vi "Reproductor de musica.vi"() -> ()   [LabVIEW 2023]
uses:
  <vilib>/Analysis/3filter.llb/Filter Passband Type.ctl
  <vilib>/express/express analysis/Spectral/Block/exnSpectralBlock spectral measurements power poly.vi
  <vilib>/express/express analysis/Spectral/XNode/ExpressSpectralMeasurementsBlockNode.xnode
  <vilib>/measure/mamon.llb/Waveform Peak Detection for 1 Chan.vi
  <vilib>/express/express analysis/Spectral/Block/exnSpectralBlock spectral measurements power WFM.vi
  <vilib>/Analysis/3filter.llb/Butterworth Filter (DBL).vi
  <vilib>/Waveform/WDTOps.llb/WDT Get Waveform Subset DBL.vi
  <vilib>/Waveform/WDTOps.llb/WDT Number of Waveform Samples DBL.vi
  <vilib>/Waveform/WDTOps.llb/WDT Waveform Duration DBL.vi
  <vilib>/Analysis/NI_AALBase.lvlib
  <vilib>/measure/NI_MAPro.lvlib
  <vilib>/Analysis/NI_AALPro.lvlib
  <vilib>/measure/NI_MABase.lvlib
panel:
  in  "phase baja \nsin filtro":dbl
  in  "Señal baja frec":T1(ring)
  in  "phase alta \nsin filtro":dbl format="%.2p"
  in  "señal alta frec":T1(ring)
  in  "señal baja frec filtrada":T1(ring)
  in  "phase bajas \nfiltro":dbl
  in  "phase altas\nfiltro":dbl format="%.2p"
  in  "señal alta frec filtrada":T1(ring)
  in  "Frecuencia \nmanual baja":dbl=10.0 format="%0.2p"
  in  "Frecuencia \nmanual alta":dbl=10.0 format="%0.2p"
  in  "tipo onda\nmanual bajas":T1(ring)
  in  "phase baja \nmanual":dbl(knob) scale=0.0..360.0
  in  "Tipo onda\nmanual altas":T1(ring)
  in  "Phase alta \nmanual":dbl(knob) scale=0.0..360.0
  in  "banda 2":dbl
  in  "banda 1":dbl
  in  "alpha":dbl
  in  "peaks/valleys 2":u16(ring) items=["Peaks", "Valleys"]
  in  "Apagado":bool
  in  "duration":dbl=1.0 format="%0.2f"
  in  "path":path
  out "Formas de onda":waveform(dbl)[](graph)
  out "Señal Adquirida 2":waveform(dbl)[](graph)
  out "sampling info":cluster{"Fs":dbl, "#s":dbl}={"Fs"=22050.0, "#s"=22050.0}
  out "Lissajous":cluster{"Array":dbl[], "Array":dbl[]}[](graph)
  out "Espectro Amplitud":cluster{"f0":dbl, "df":dbl, "magnitude":dbl[]}(graph)
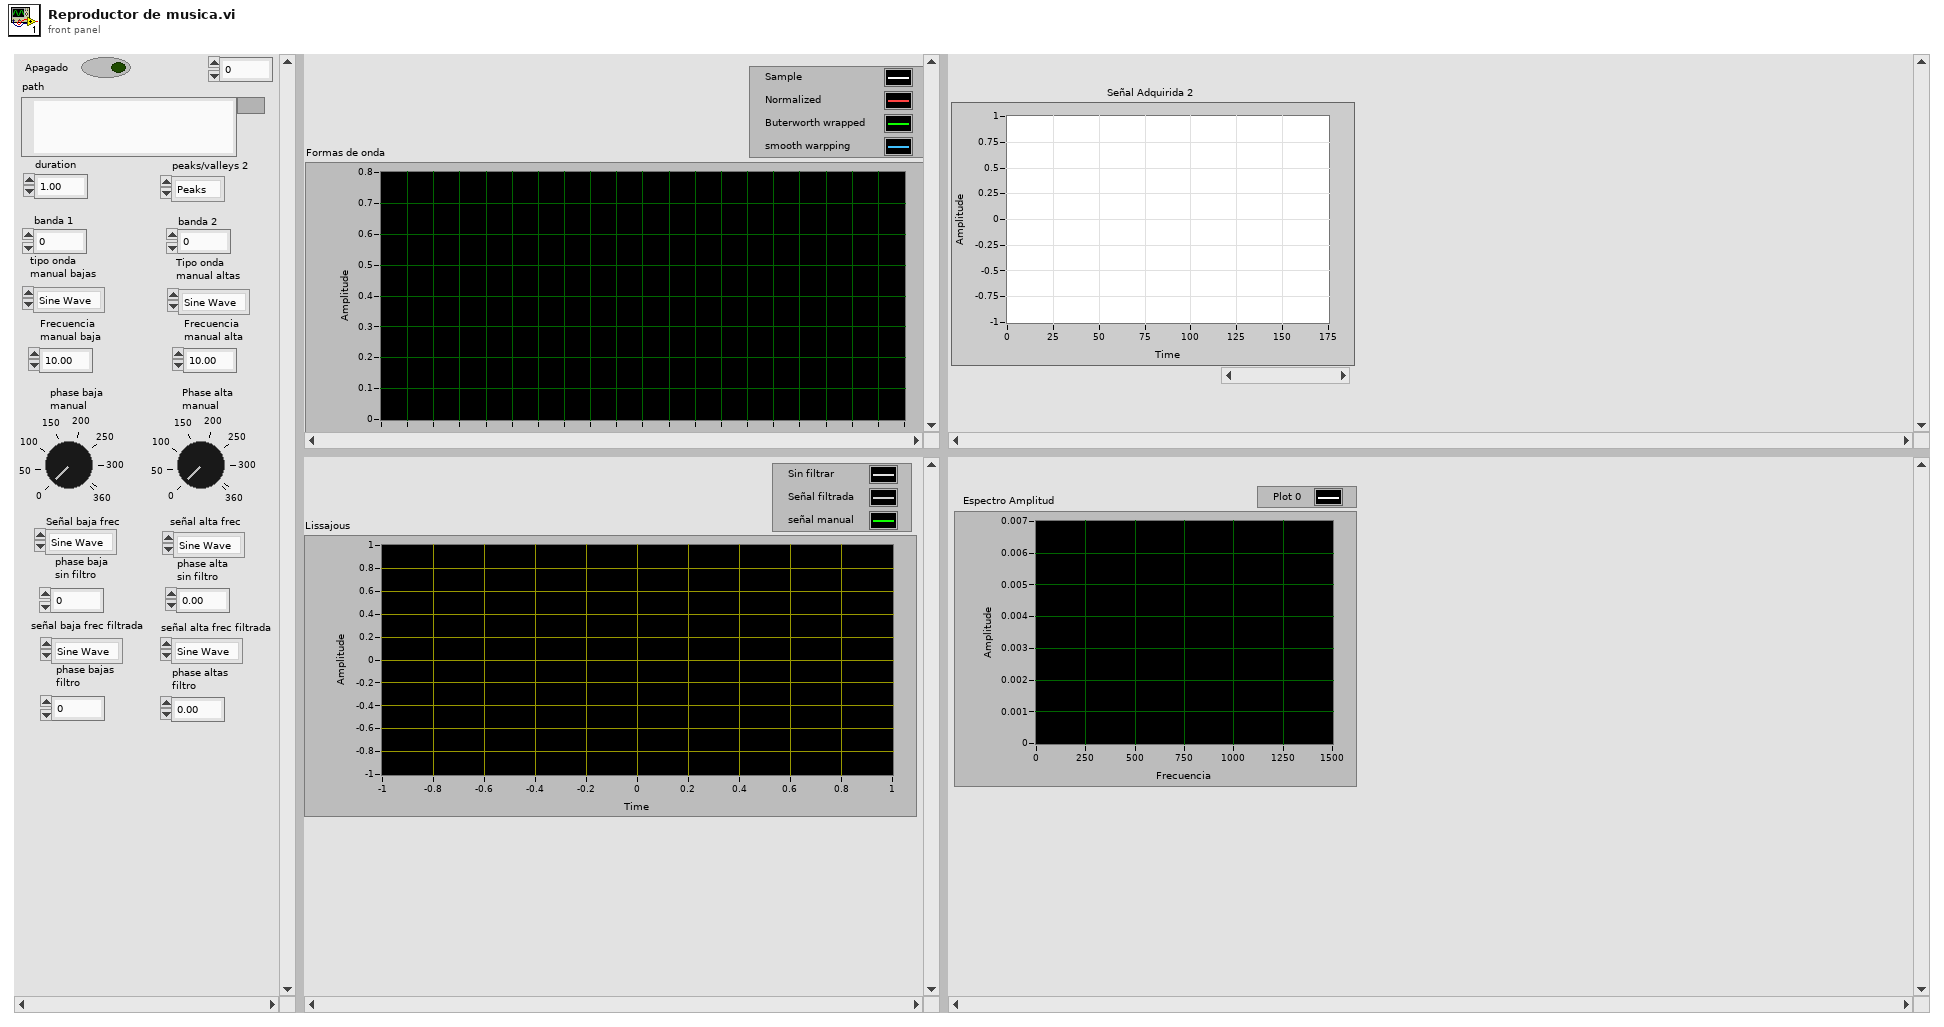
[diagram p1: front panel]
types:
  T1 = enum16{"Sine Wave", "Triangle Wave", "Square Wave", "Sawtooth Wave"}
  T2 = typedef "NI_AALBase.lvlib/Filter Passband Type.ctl" = enum32{"Lowpass", "Highpass", "Bandpass", "Bandstop"}
  T3 = cluster{"averaging mode":u16, "weighting mode":u16, "number of averages":u32}
  T4 = cluster{"dB On (F)":bool, "unwrap phase (F)":bool, "convert to degree (F)":bool}
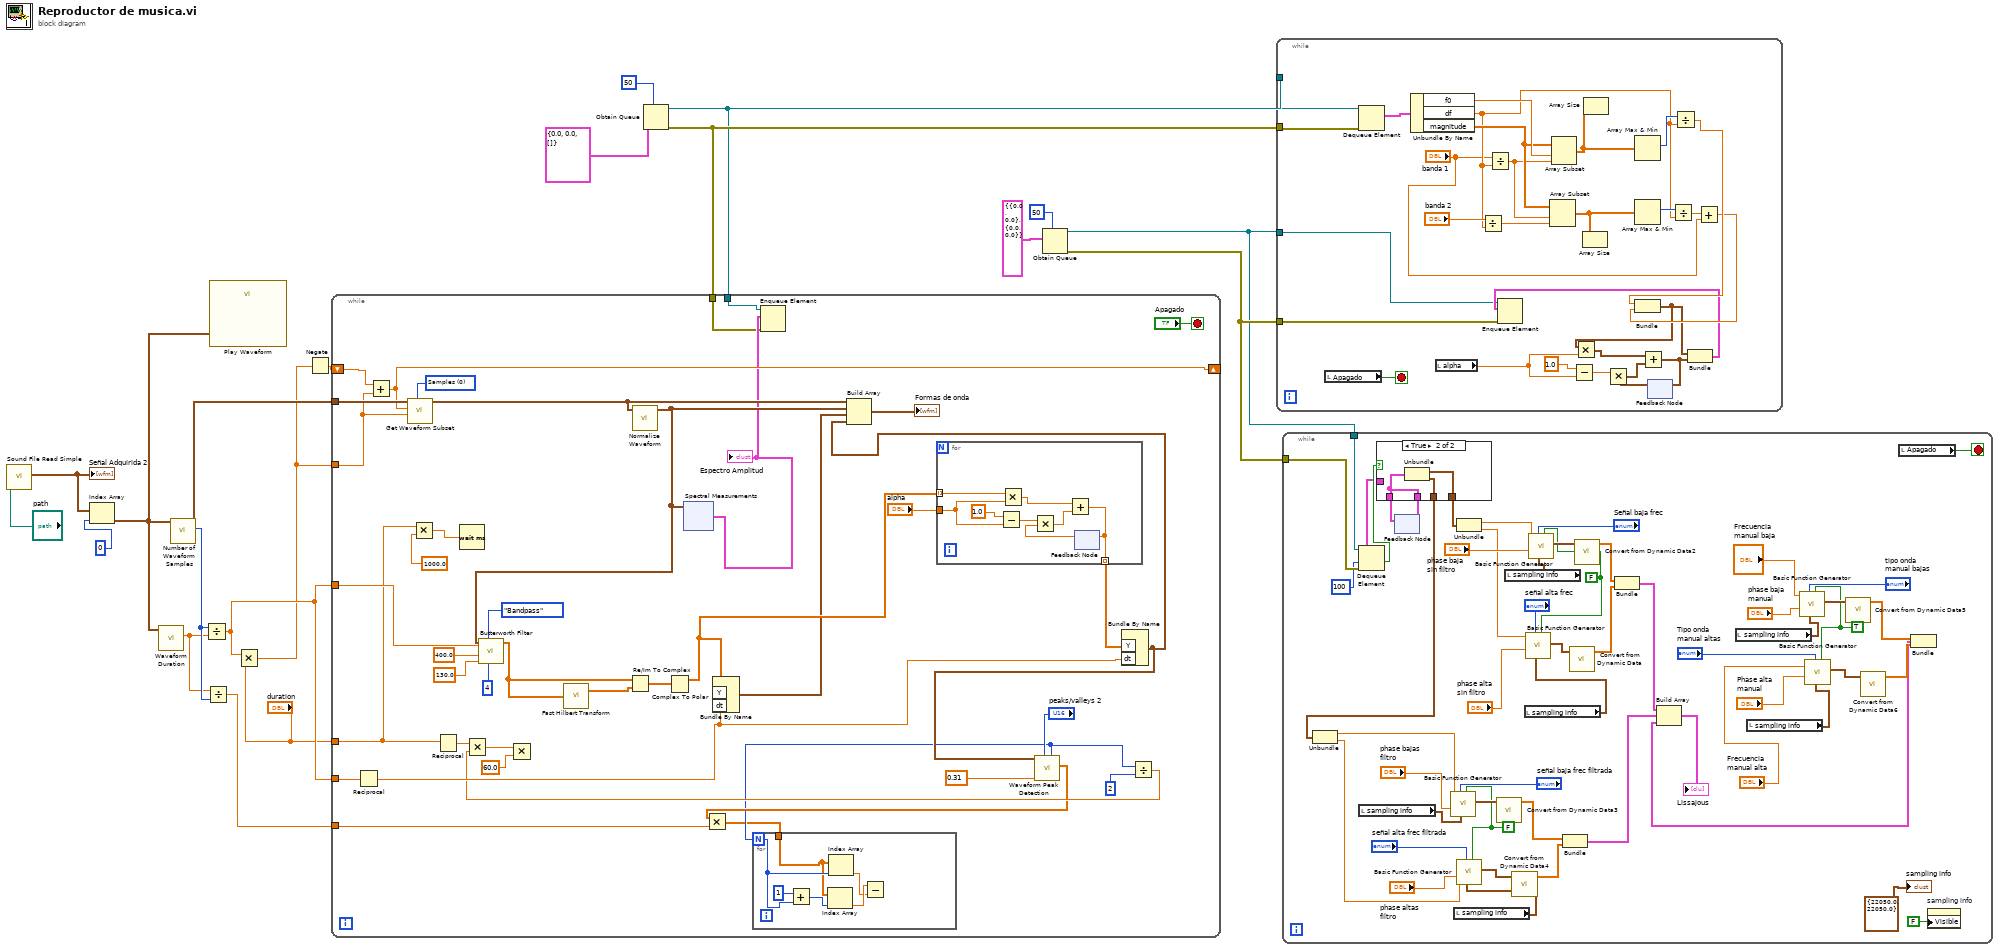
[diagram p0: block diagram]
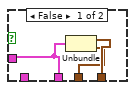
[diagram p2: hidden frame]
diagram:
  n1 = call <vilib>:"Sound File Read Simple.vi"("path"="path") -> ("data"=w19:waveform(dbl)[])  [unwired: 7 in, 3 out]
  "Señal Adquirida 2" <- w19
  n2 = Index Array(array=w19, index=0) -> (element=w10:waveform(dbl))
  n3 = call-poly <vilib>:"Waveform Duration.vi"("waveform in"=w10) -> ("duration"=w15:dbl)  [unwired: 8 in, 2 out]
  n4 = call-poly <vilib>:"Number of Waveform Samples.vi"("waveform in"=w10) -> ("number of samples"=w17:i32, "waveform out"=w16:waveform(dbl))  [unwired: 8 in, 1 out]
  n5 = Divide(x=w17, y=w15) -> (x/y=w13:dbl)
  n6 = Divide(x=w15, y=w17) -> (x/y=w14:dbl)
  n7 = call "Play Waveform"("Data"=w10) -> ()  [unwired: 18 in, 1 out]
  n8 = Multiply(x=w13, y="duration") -> (x*y=w12:dbl)
  n9 = Negate(x=w12) -> (-x=w11:dbl)
  n10 = Obtain Queue(max queue size (-1, unlimited)=50, element data type=cluster{"f0":dbl, "df":dbl, "magnitude":dbl[]} {"f0"=0.0, "df"=0.0, "magnitude"=[]} ("Power Spectrum")) -> (queue out=w4:refnum<queue>, error out=w7:errorcluster)  [unwired: 3 in, 1 out]
  n11 = while {
    tunnel: w16 -> [w35]
    tunnel: w14 -> [w34]
    tunnel: w13 -> [w33]
    shift-right: [w25] -> _
    shift-left: w11 -> [w26]
    tunnel: w13 -> [w29]
    tunnel: "duration" -> [w28]
    tunnel: w12 -> [w27]
    tunnel: w7 -> [w22]
    tunnel: w4 -> [w21]
    stop <- "Apagado" stop-if-true
    w30 = u16 0 items=["Samples", "Relative Time"] ("start/duration format")
    n12 = Reciprocal(x=w29) -> (1/x=w45:dbl)
    n13 = Add(x=w26, y=w27) -> (x+y=w25:dbl)
    n14 = call-poly <vilib>:"Get Waveform Subset.vi"("start/duration format"=w30, "duration"=w27, "start samples/time"=w25, "waveform in"=w35) -> ("waveform out"=w24:waveform(dbl))  [unwired: 2 in, 3 out]
    n15 = Multiply(x=w28, y=1000.0) -> (x*y=w32:dbl)
    n16 = Reciprocal(x=w28) -> (1/x=w42:dbl)
    n17 = Wait (ms)(milliseconds to wait=w32) -> ()  [unwired: 1 out]
    n18 = call <vilib>:"Normalize Waveform.vi"("waveform in"=w24) -> ("normalized waveform"=w56:waveform(dbl))  [unwired: 7 in, 3 out]
    n19 = call-poly <vilib>:"Butterworth Filter.vi"("order"=4, "filter type"=Filter_Passband_Type."Bandpass", "low cutoff freq: fl"=130.0, "high cutoff freq: fh"=400.0 ("low cutoff freq: fl"), "sampling freq: fs"=w33, "X"=w56) -> ("Filtered X"=w51:dbl[])  [unwired: 2 in, 1 out]
    n20 = call <vilib>:"Fast Hilbert Transform.vi"("X"=w51) -> ("Hilbert{X}"=w52:dbl[])  [unwired: 1 out]
    n21 = Re/Im To Complex(1:w52, 2:w51) -> (0:w50:cdb[])
    n22 = Complex To Polar(r * e^(i*theta)=w50) -> (r=w48:dbl[])  [unwired: 1 out]
    n23 = xnode "Spectral Measurements"("Signals"=w56) -> ("Power Spectrum"=w23:cluster{"f0":dbl, "df":dbl, "magnitude":dbl[]})  [unwired: 1 in, 1 out]
    "Espectro Amplitud" <- w23
    n24 = Bundle By Name("Y"=w48, "dt"=w45) -> (w36:waveform(dbl))  [unwired: 1 in]
    n25 = Enqueue Element(queue=w21, element=w23, error in (no error)=w22) -> ()  [unwired: 4 out]
    n26 = for {
      tunnel: "alpha" -> [w74]
      tunnel: w48 -> [w69] mode=indexing
      tunnel: [w68] -> w47 mode=indexing
      n27 = Subtract(x=1.0, y=w74) -> (x-y=w73:dbl)
      n28 = Multiply(x=w69, y=w74) -> (x*y=w71:dbl)
      n29 = feedback #1() -> (w70:dbl)  [unwired: 1 in]
      n30 = Multiply(x=w73, y=w70) -> (x*y=w72:dbl)
      n31 = Add(x=w71, y=w72) -> (x+y=w68:dbl)
      n32 = feedback-in #1(w68) -> ()
    }
    n33 = Bundle By Name("Y"=w47, "dt"=w45) -> (w46:waveform(dbl))  [unwired: 1 in]
    n34 = Build Array(w24, w56, w36, w46) -> (→"Formas de onda":waveform(dbl)[])
    n35 = call-poly <vilib>:"Waveform Peak Detection.vi"("peaks/valleys"="peaks/valleys 2", "threshold"=0.31, "Signal In"=w46) -> ("Locations"=w39:dbl[], "# found"=w38:i32)  [unwired: 4 in, 3 out]
    n36 = Multiply(x=w39, y=w34) -> (x*y=w37:dbl[])
    n37 = for {
      N: w38 -> [w65]
      tunnel: w37 -> [w64]
      n38 = Add(x=1 ("index"), y=w65) -> (x+y=w66:i32)
      n39 = Index Array(array=w64, index=w66) -> (element=w63:dbl)
      n40 = Index Array(array=w64, index=w65) -> (element=w62:dbl)
      n41 = Subtract(x=w63, y=w62) -> ()  [unwired: 1 out]
    }
    n42 = Divide(x=w38, y=2 ("threshold")) -> (x/y=w43:dbl)
    n43 = Multiply(x=w42, y=w43) -> (x*y=w41:dbl)
    n44 = Multiply(x=w41, y=60.0 ("low cutoff freq: fl")) -> ()  [unwired: 1 out]
  }
  n45 = Obtain Queue(max queue size (-1, unlimited)=50, element data type=cluster{cluster{dbl, dbl}, cluster{dbl, dbl}} {{0.0, 0.0}, {0.0, 0.0}} ("output cluster")) -> (queue out=w2:refnum<queue>, error out=w3:errorcluster)  [unwired: 3 in, 1 out]
  n46 = while {
    tunnel: w2 -> [w85]
    tunnel: w3 -> [w86]
    tunnel: w4 -> [w91]
    tunnel: w7 -> [w90]
    stop <- w87 stop-if-true
    n47 = local read "Apagado"() -> (w87:bool)
    n48 = Dequeue Element(queue=w91, error in (no error)=w90) -> (element=w89:cluster{"f0":dbl, "df":dbl, "magnitude":dbl[]})  [unwired: 4 out]
    n49 = Unbundle By Name(w89) -> ("f0"=w113:dbl, "df"=w103:dbl, "magnitude"=w111:dbl[])
    n50 = local read "alpha"() -> (w88:dbl)
    n51 = Divide(x="banda 2", y=w103) -> (x/y=w112:dbl)
    n52 = Divide(x="banda 1", y=w103) -> (x/y=w108:dbl)
    n53 = Array Subset(array=w111, index=w108, length=w112) -> (w107:dbl[])
    n54 = Array Subset(array=w111, index=w113, length=w108) -> (w109:dbl[])
    n55 = Subtract(x=1.0, y=w88) -> (x-y=w99:dbl)
    n56 = Array Size(array=w107) -> ()  [unwired: 1 out]
    n57 = Array Size(array=w109) -> ()  [unwired: 1 out]
    n58 = Array Max & Min(array=w109) -> (max index (indices)=w106:i32)  [unwired: 3 out]
    n59 = Array Max & Min(array=w107) -> (max index (indices)=w105:i32)  [unwired: 3 out]
    n60 = feedback #2() -> (w96:cluster{dbl, dbl})  [unwired: 1 in]
    n61 = Multiply(x=w99, y=w96) -> (x*y=w98:cluster{dbl, dbl})
    n62 = Divide(x=w105, y=w103) -> (x/y=w104:dbl)
    n63 = Divide(x=w106, y=w103) -> (x/y=w102:dbl)
    n64 = Add(x=w104, y="banda 1") -> (x+y=w101:dbl)
    n65 = Bundle(w102, w101) -> (w95:cluster{dbl, dbl})  [unwired: 1 in]
    n66 = Multiply(x=w95, y=w88) -> (x*y=w97:cluster{dbl, dbl})
    n67 = Add(x=w97, y=w98) -> (x+y=w94:cluster{dbl, dbl})
    n68 = feedback-in #2(w94) -> ()
    n69 = Bundle(w95, w94) -> (w93:cluster{cluster{dbl, dbl}, cluster{dbl, dbl}})  [unwired: 1 in]
    n70 = Enqueue Element(queue=w85, element=w93, error in (no error)=w86) -> ()  [unwired: 4 out]
  }
  n71 = while {
    tunnel: w2 -> [w160]
    tunnel: w3 -> [w159]
    stop <- w122 stop-if-true
    w127 = TRUE ("reset signal")
    w137 = FALSE ("reset signal")
    w139 = FALSE ("reset signal")
    n72 = Dequeue Element(queue=w160, timeout in ms (-1)=100, error in (no error)=w159) -> (element=w142:cluster{cluster{dbl, dbl}, cluster{dbl, dbl}}, timed out?=w146:bool)  [unwired: 2 out]
    n73 = local read "sampling info"() -> (w116:cluster{"Fs":dbl, "#s":dbl})
    n74 = feedback #3() -> (w143:cluster{cluster{dbl, dbl}, cluster{dbl, dbl}})  [unwired: 1 in]
    n75 = case shown="True" w146 {
      tunnel: [w171 w174] -> w145
      tunnel: [w170 w173] -> w144
      tunnel: w143 -> [_ w172]
      tunnel: w142 -> [w169 _]
      tunnel: [w169 w172] -> w141
      frame False {
        n76 = Unbundle(w169) -> (w171:cluster{dbl, dbl}, w170:cluster{dbl, dbl})
      }
      frame True {
        n77 = Unbundle(w172) -> (w174:cluster{dbl, dbl}, w173:cluster{dbl, dbl})
      }
    }
    n78 = Unbundle(w144) -> (w136:dbl, w135:dbl)
    n79 = feedback-in #3(w141) -> ()
    n80 = call <vilib>:"Basic Function Generator.vi"("reset signal"=w139, "sampling info"=w116, "signal type"="señal baja frec filtrada", "phase"="phase bajas \nfiltro", "frequency"=w136) -> ("signal out"=w157:waveform(dbl))  [unwired: 4 in, 2 out]
    n81 = local read "sampling info"() -> (w117:cluster{"Fs":dbl, "#s":dbl})
    n82 = Unbundle(w145) -> (w158:dbl, w149:dbl)
    n83 = call <vilib>:"Basic Function Generator.vi"("reset signal"=w139, "sampling info"=w117, "signal type"="señal alta frec filtrada", "phase"="phase altas\nfiltro", "frequency"=w135) -> ("signal out"=w154:waveform(dbl))  [unwired: 4 in, 2 out]
    n84 = call "Convert from Dynamic Data3"("Dynamic Data Type"=w157) -> ("Array"=w152:dbl[])  [unwired: 3 in]
    n85 = local read "sampling info"() -> (w115:cluster{"Fs":dbl, "#s":dbl})
    n86 = call "Convert from Dynamic Data4"("Dynamic Data Type"=w154) -> ("Array"=w140:dbl[])  [unwired: 3 in]
    n87 = local read "sampling info"() -> (w114:cluster{"Fs":dbl, "#s":dbl})
    n88 = call <vilib>:"Basic Function Generator.vi"("reset signal"=w137, "sampling info"=w114, "signal type"="señal alta frec", "phase"="phase alta \nsin filtro", "frequency"=w149) -> ("signal out"=w165:waveform(dbl))  [unwired: 4 in, 2 out]
    n89 = call <vilib>:"Basic Function Generator.vi"("reset signal"=w137, "sampling info"=w115, "signal type"="Señal baja frec", "phase"="phase baja \nsin filtro", "frequency"=w158) -> ("signal out"=w166:waveform(dbl))  [unwired: 4 in, 2 out]
    n90 = Bundle("Array"=w152, "Array"=w140) -> (w138:cluster{"Array":dbl[], "Array":dbl[]})  [unwired: 1 in]
    n91 = call "Convert from Dynamic Data"("Dynamic Data Type"=w165) -> ("Array"=w167:dbl[])  [unwired: 3 in]
    n92 = call "Convert from Dynamic Data2"("Dynamic Data Type"=w166) -> ("Array"=w168:dbl[])  [unwired: 3 in]
    n93 = Bundle("Array"=w168, "Array"=w167) -> (w151:cluster{"Array":dbl[], "Array":dbl[]})  [unwired: 1 in]
    n94 = local read "sampling info"() -> (w118:cluster{"Fs":dbl, "#s":dbl})
    n95 = local read "sampling info"() -> (w119:cluster{"Fs":dbl, "#s":dbl})
    n96 = call <vilib>:"Basic Function Generator.vi"("reset signal"=w127, "sampling info"=w118, "signal type"="tipo onda\nmanual bajas", "phase"="phase baja \nmanual", "frequency"="Frecuencia \nmanual baja") -> ("signal out"=w134:waveform(dbl))  [unwired: 4 in, 2 out]
    n97 = call <vilib>:"Basic Function Generator.vi"("reset signal"=w127, "sampling info"=w119, "signal type"="Tipo onda\nmanual altas", "phase"="Phase alta \nmanual", "frequency"="Frecuencia \nmanual alta") -> ("signal out"=w131:waveform(dbl))  [unwired: 4 in, 2 out]
    n98 = call "Convert from Dynamic Data5"("Dynamic Data Type"=w134) -> ("Array"=w130:dbl[])  [unwired: 3 in]
    n99 = call "Convert from Dynamic Data6"("Dynamic Data Type"=w131) -> ("Array"=w128:dbl[])  [unwired: 3 in]
    n100 = local read "Apagado"() -> (w122:bool)
    n101 = Bundle("Array"=w130, "Array"=w128) -> (w124:cluster{"Array":dbl[], "Array":dbl[]})  [unwired: 1 in]
    n102 = Build Array(w151, w138, w124) -> (→"Lissajous":cluster{"Array":dbl[], "Array":dbl[]}[])
    n103 = property on="sampling info" class="Clust (strict)"("Visible"=FALSE) -> ()  [unwired: 2 in, 2 out]
    "sampling info" <- cluster{"Fs":dbl, "#s":dbl} {"Fs"=22050.0, "#s"=22050.0} ("sampling info")
  }
